vi "Write First Header Contents Class Array .vi"(8 "error in (no error)":errorcluster, 10 "Header Contents.lvclass":refnum<class "Header Contents.lvclass">, 11 "Simulated_Header in":refnum<class "Simulated_Header.lvclass">) -> (0 "error out":errorcluster, 3 "Simulated_Header out":refnum<class "Simulated_Header.lvclass">)   [LabVIEW 2018, in "Simulated_Header.lvclass"]
uses:
  Simulated_Header.lvclass
  Header Contents/Header Contents.lvclass
  Simulated_Header.lvclass/Simulated_Header.ctl
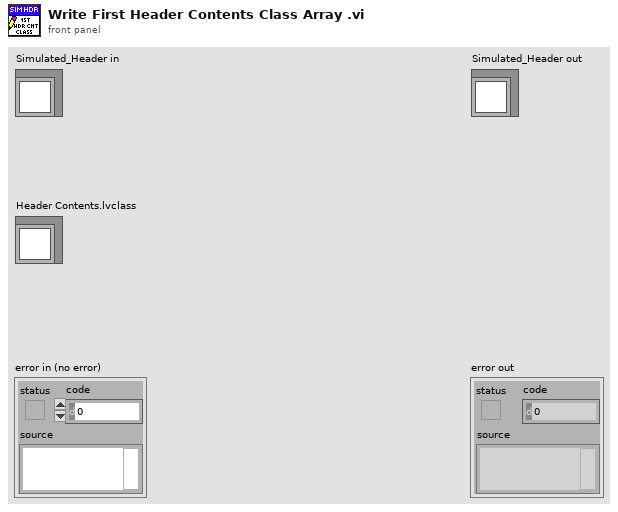
[diagram p1: front panel]
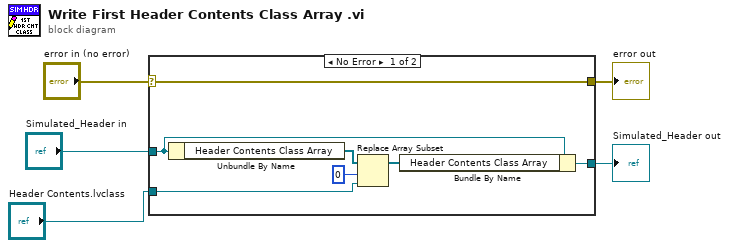
[diagram p0: block diagram]
diagram:
  n1 = case shown="No Error" "error in (no error)" {
    selector: "error in (no error)" -> [w12 w13]
    tunnel: [w12 w13] -> w4
    tunnel: [w11 w14] -> w2
    tunnel: "Simulated_Header in" -> [w10 w14]
    tunnel: "Header Contents.lvclass" -> [w8 _]
    frame No Error {
      n2 = Unbundle By Name(w10) -> ("Header Contents Class Array"=w7:refnum<class "Header Contents.lvclass">[])
      n3 = Replace Array Subset(array=w7, new element=w8, index=0) -> (w9:refnum<class "Header Contents.lvclass">[])
      n4 = Bundle By Name(cluster=w10, "Header Contents Class Array"=w9) -> (w11:refnum<class "Simulated_Header.lvclass">)
    }
    frame Error {
    }
  }
  "error out" <- w4
  "Simulated_Header out" <- w2
